vi "FTW-JSON-ObjectManip-GetPair-Integer.vi"(0 "Input JSON Object":string, 5 "Key":string, 7 "Default Value":i64, 9 "Consume Value":bool, 11 "error in":errorcluster) -> (4 "Output JSON Object":string, 8 "Value":i64, 10 "Found":bool, 15 "error out":errorcluster)   [LabVIEW 2015]
panel:
  # "Inputs"
  # "Outputs"
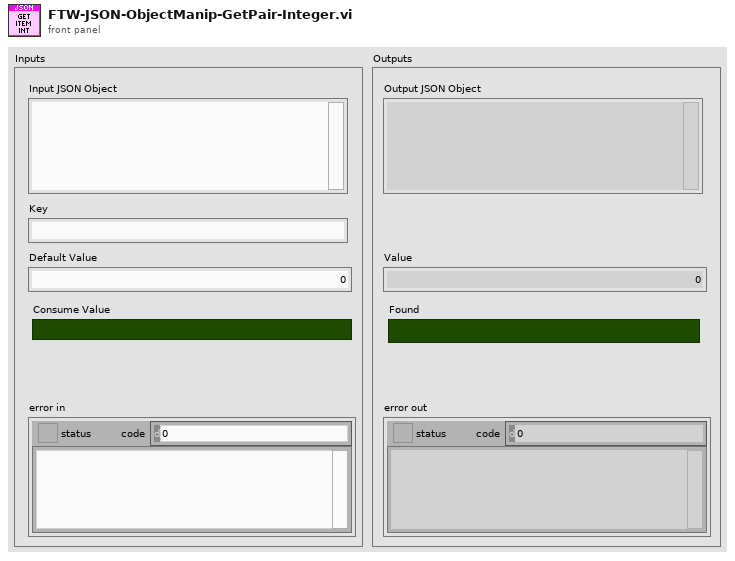
[diagram p1: front panel]
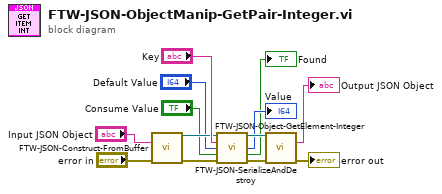
[diagram p0: block diagram]
diagram:
  n1 = call "FTW-JSON-Construct-FromBuffer.vi"("JSON String (UTF-8)"="Input JSON Object", "error in"="error in") -> ("JSON"=w10:refnum<class "FTW-Container.lvclass">, "error out"=w8:errorcluster)  [unwired: 12 in]
  n2 = call "FTW-JSON-Object-GetElement-Integer.vi"("JSON"=w10, "Key"="Key", "Default Value"="Default Value", "Consume Value"="Consume Value", "error in"=w8) -> ("JSON out"=w9:refnum<class "FTW-Container.lvclass">, "Value"=→"Value":i64, "Found"=→"Found":bool, "error out"=w7:errorcluster)  [unwired: 6 in, 1 out]
  n3 = call "FTW-JSON-SerializeAndDestroy.vi"("JSON"=w9, "error in"=w7) -> ("JSON String (UTF-8)"=→"Output JSON Object":string, "error out"=→"error out":errorcluster)  [unwired: 12 in]
